vi "Read Element of Max Current Limit.vi"(8 "error in (no error)":errorcluster, 10 "index":i32, 11 "CS++DCPwrChannelData in":refnum<class "CS++DCPwrChannelData.lvclass">) -> (0 "error out":errorcluster, 2 "max current limit":dbl[unit] format="%^.2e", 3 "CS++DCPwrChannelData out":refnum<class "CS++DCPwrChannelData.lvclass">)   [LabVIEW 2016, in "CS++DCPwrGui.lvlib" / "CS++DCPwrChannelData.lvclass"]
uses:
  CS++DCPwrChannelData.lvclass
  CS++DCPwrChannelData.lvclass/CS++DCPwrChannelData.ctl
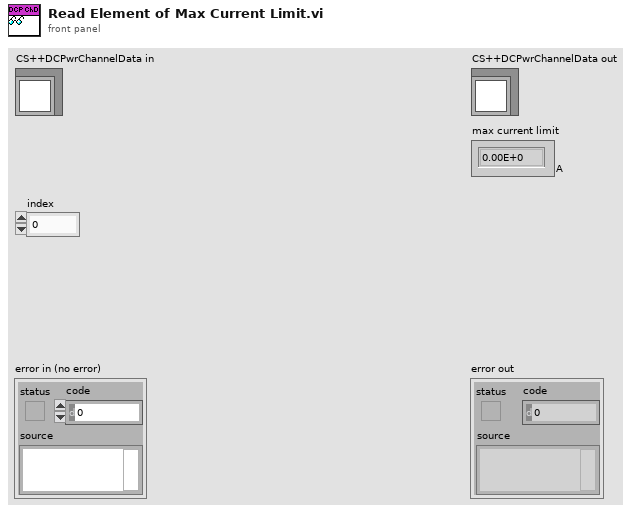
[diagram p1: front panel]
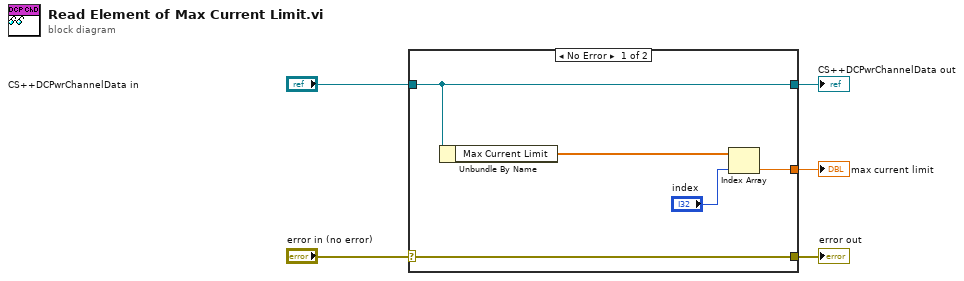
[diagram p0: block diagram]
diagram:
  n1 = case shown="No Error" "error in (no error)" {
    selector: "error in (no error)" -> [w10 w11]
    tunnel: [w10 w11] -> w4
    tunnel: [w9 w12] -> w2
    tunnel: "CS++DCPwrChannelData in" -> [w9 w12]
    tunnel: [w6 _] -> w1
    frame No Error {
      n2 = Unbundle By Name(w9) -> ("Max Current Limit"=w8:dbl[unit][])
      n3 = Index Array(array=w8, index="index") -> (element=w6:dbl[unit])
    }
    frame Error {
    }
  }
  "error out" <- w4
  "CS++DCPwrChannelData out" <- w2
  "max current limit" <- w1
